vi "JSON to Framework Configuration.vi"(8 "error in (no error)":errorcluster, 10 "JSON string":string, 11 "JSON Builder in":refnum<class "JSON Builder.lvclass">) -> (0 "error out":errorcluster, 2 "Framework Configuration":T1, 3 "JSON Builder out":refnum<class "JSON Builder.lvclass">)   [LabVIEW 2017, in "DSF Core.lvlib" / "JSON Builder.lvclass"]
uses:
  JSON Builder.lvclass
  Typedefs/DSF Engine Framework Configuration.ctl
  Typedefs/DSF Engine Plugin Configuration.ctl
  Typedefs/DSF Timing Info.ctl
  Typedefs/DSF Engine Plugin Thread Configuration.ctl
  Typedefs/DSF Settings Info.ctl
  Typedefs/DSF Engine Transfer Group Configuration.ctl
  Typedefs/DSF Direction.ctl
  Typedefs/DSF Engine Transfer Configuration.ctl
  Typedefs/DSF Byte Order.ctl
  Typedefs/DSF Engine Channel Configuration.ctl
  Typedefs/DSF Data Type.ctl
  Typedefs/DSF Timeout Behavior.ctl
  Typedefs/DSF Engine Framework JSON Configuration.ctl
  Typedefs/DSF Engine Plugin JSON Configuration.ctl
  Typedefs/DSF Engine Transfer Group JSON Configuration.ctl
  Typedefs/DSF Engine Transfer JSON Configuration.ctl
  Typedefs/DSF Engine Channel JSON Configuration.ctl
  DSF Core.lvlib
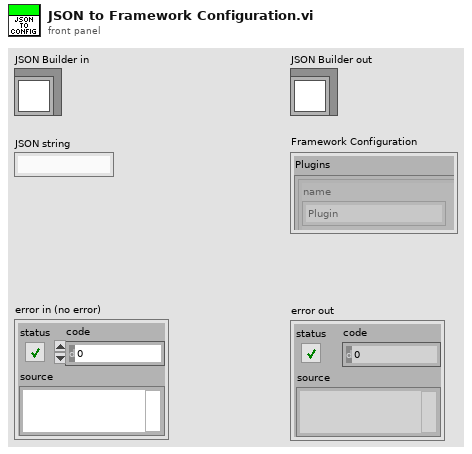
[diagram p1: front panel]
types:
  T1 = typedef "DSF Core.lvlib/DSF Engine Framework Configuration.ctl" = cluster{"Plugins":T2[]}
  T2 = typedef "DSF Core.lvlib/DSF Engine Plugin Configuration.ctl" = cluster{"name":string, "components":string[], "cycle timing":T3, "threads":T4[], "Transfer Groups":T6[], "settings":T5}
  T3 = typedef "DSF Core.lvlib/DSF Timing Info.ctl" = cluster{"priority":u64, "decimation":u64, "offset":u64}
  T4 = typedef "DSF Core.lvlib/DSF Engine Plugin Thread Configuration.ctl" = cluster{"buffer converter settings":T5, "transceiver settings":T5, "custom settings":T5, "processor":i32, "priority offset":i16}
  T5 = typedef "DSF Core.lvlib/DSF Settings Info.ctl" = cluster{"key":string, "value":string}[]
  T6 = typedef "DSF Core.lvlib/DSF Engine Transfer Group Configuration.ctl" = cluster{"name":string, "direction":T7, "cycle timing":T3, "thread index":i32, "settings":T5, "Transfers":T8[], "timeout behavior":T12}
  T7 = typedef "DSF Core.lvlib/DSF Direction.ctl" = enum8{"Tx", "Rx"}
  T8 = typedef "DSF Core.lvlib/DSF Engine Transfer Configuration.ctl" = cluster{"name":string, "byte order":T9, "settings":T5, "channels":T10[]}
  T9 = typedef "DSF Core.lvlib/DSF Byte Order.ctl" = enum8{"big-endian", "little-endian"}
  T10 = typedef "DSF Core.lvlib/DSF Engine Channel Configuration.ctl" = cluster{"string offset":u64, "string data type":T11, "engine data type":T11, "name":string, "settings":T5, "units":string}
  T11 = typedef "DSF Core.lvlib/DSF Data Type.ctl" = enum8{"Bool", "SGL", "DBL", "I8", "I16", "I32", "I64", "U8", "U16", "U32", "U64"}
  T12 = typedef "DSF Core.lvlib/DSF Timeout Behavior.ctl" = enum8{"Increment Late Count", "Throw Error"}
  T13 = typedef "DSF Core.lvlib/JSON Builder.lvclass/DSF Engine Framework JSON Configuration.ctl" = cluster{"Plugins":T14[]}
  T14 = typedef "DSF Core.lvlib/JSON Builder.lvclass/DSF Engine Plugin JSON Configuration.ctl" = cluster{"name":string, "components":string[], "cycle timing":T3, "threads":T4[], "Transfer Groups":T15[], "settings":T5}
  T15 = typedef "DSF Core.lvlib/JSON Builder.lvclass/DSF Engine Transfer Group JSON Configuration.ctl" = cluster{"name":string, "direction":u8, "cycle timing":T3, "thread index":i32, "settings":T5, "Transfers":T16[], "timeout behavior":u8}
  T16 = typedef "DSF Core.lvlib/JSON Builder.lvclass/DSF Engine Transfer JSON Configuration.ctl" = cluster{"name":string, "byte order":u8, "settings":T5, "channels":T17[]}
  T17 = typedef "DSF Core.lvlib/JSON Builder.lvclass/DSF Engine Channel JSON Configuration.ctl" = cluster{"string offset":u64, "string data type":u8, "engine data type":u8, "name":string, "settings":T5, "units":string}
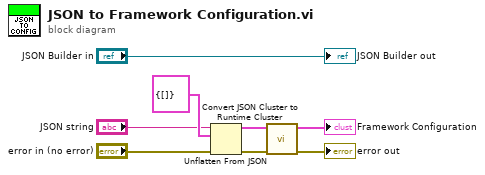
[diagram p0: block diagram]
diagram:
  n1 = Unflatten From JSON(JSON string="JSON string", type and defaults=T13 {"Plugins"=[]} ("Framework Configuration"), error in (no error)="error in (no error)") -> (value=w6:T13, error out=w7:errorcluster)  [unwired: 4 in]
  n2 = call "Convert JSON Cluster to Runtime Cluster.vi"("error in (no error)"=w7, "Framework JSON Configuration"=w6) -> ("error out"=→"error out":errorcluster, "Framework Configuration"=→"Framework Configuration":T1)  [unwired: 8 in]
  "JSON Builder out" <- "JSON Builder in"
